vi "FoodCountDown.vi"(10 "Food time in":u16[][](array[numeric]), 11 "Map in":u16[][](array[numeric])) -> (2 "Array 2":u16[][](array[numeric]), 3 "Array":u16[][](array[numeric]))   [LabVIEW 2014]
doc: "Count down for each food."
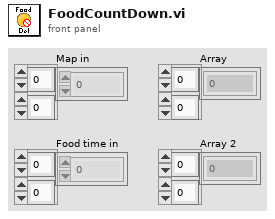
[diagram p1: front panel]
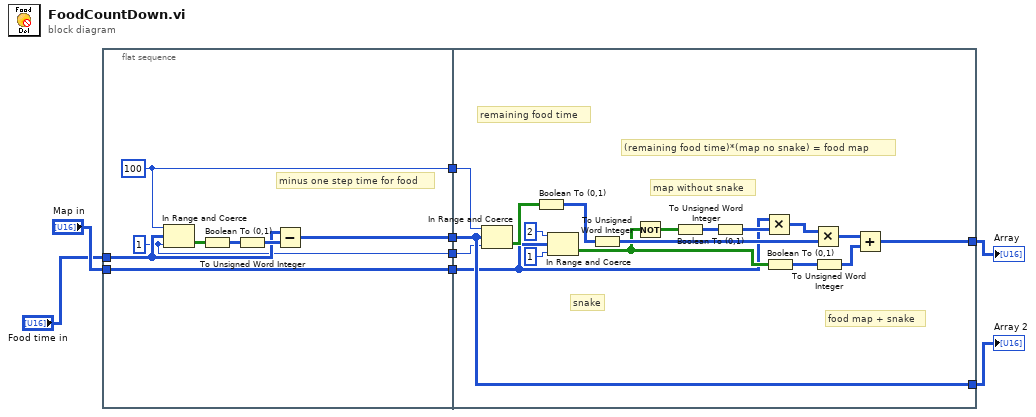
[diagram p0: block diagram]
diagram:
  n1 = flat-sequence {
    tunnel: "Food time in" -> [w13]
    tunnel: "Map in" -> [w11]
    tunnel: [w12] -> w8
    tunnel: [w11] -> w7
    tunnel: [w10] -> w6
    tunnel: [w9] -> w5
    tunnel: [w30] -> w2
    tunnel: w8 -> [w30]
    tunnel: w7 -> [w19]
    tunnel: w6 -> [w26]
    tunnel: w5 -> [w27]
    tunnel: [w17] -> w4
    frame #0 {
      w10 = u16 100
      w9 = u16 1
      # "minus one step time for food"
      n2 = In Range and Coerce(upper limit=w10, x=w13, lower limit=w9) -> (In Range?=w15:bool[][])  [unwired: 1 out]
      n3 = Boolean To (0,1)(Boolean=w15) -> (0, 1=w16:i16[][])
      n4 = To Unsigned Word Integer(number=w16) -> (unsigned 16bit integer=w14:u16[][])
      n5 = Subtract(x=w13, y=w14) -> (x-y=w12:u16[][])
    }
    frame #1 {
      # "food map + snake"
      # "(remaining food time)*(map no snake) = food map"
      # "remaining food time"
      # "map without snake"
      # "snake"
      n6 = In Range and Coerce(upper limit=w26, x=w30, lower limit=w27) -> (In Range?=w28:bool[][])  [unwired: 1 out]
      n7 = Boolean To (0,1)(Boolean=w28) -> (0, 1=w29:i16[][])
      n8 = In Range and Coerce(upper limit=u16 2, x=w19, lower limit=u16 1) -> (In Range?=w23:bool[][])  [unwired: 1 out]
      n9 = To Unsigned Word Integer(number=w29) -> (unsigned 16bit integer=w25:u16[][])
      n10 = Not(x=w23) -> (.not. x?=w22:bool[][])
      n11 = Boolean To (0,1)(Boolean=w22) -> (0, 1=w21:i16[][])
      n12 = To Unsigned Word Integer(number=w21) -> (unsigned 16bit integer=w20:u16[][])
      n13 = Multiply(x=w19, y=w20) -> (x*y=w18:u16[][])
      n14 = Boolean To (0,1)(Boolean=w23) -> (0, 1=w33:i16[][])
      n15 = Multiply(x=w18, y=w25) -> (x*y=w34:u16[][])
      n16 = To Unsigned Word Integer(number=w33) -> (unsigned 16bit integer=w24:u16[][])
      n17 = Add(x=w34, y=w24) -> (x+y=w17:u16[][])
    }
  }
  "Array" <- w4
  "Array 2" <- w2
